vi "operationModeSelector.vi"() -> (6 "selectedMode":string, 7 "isError":bool, 8 "stopWaiting":bool)   [LabVIEW 2014]
panel:
  in  "ctrlDP":bool
  in  "ctrlManualForce":bool
  in  "ctrlManualThrusters":bool
  # "Please select an operational mode for CS Saucer"
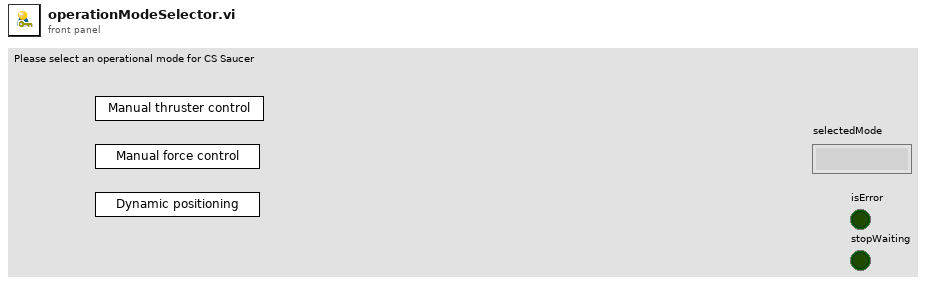
[diagram p1: front panel]
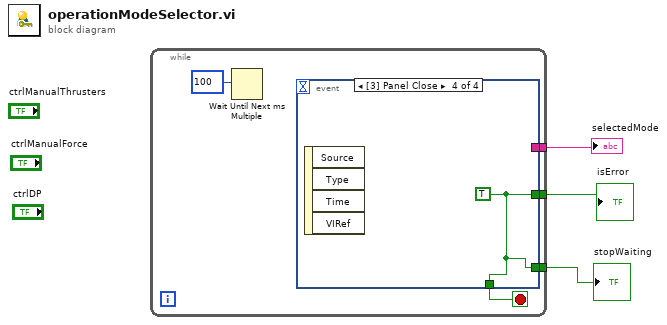
[diagram p0: block diagram]
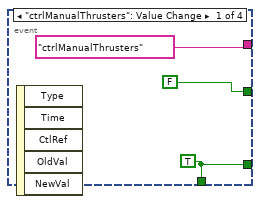
[diagram p2: hidden frame]
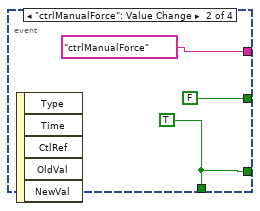
[diagram p3: hidden frame]
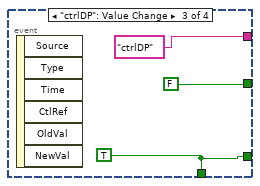
[diagram p4: hidden frame]
diagram:
  n1 = while {
    tunnel: [w8] -> w3
    tunnel: [w5] -> w2
    tunnel: [w4] -> w1
    stop <- w6 stop-if-true
    n2 = Wait Until Next ms Multiple(millisecond multiple=100) -> ()  [unwired: 1 out]
    n3 = event shown="[3] Panel Close" {
      selector: _ -> [_ _ _ _]
      dyn-events: _ -> [_ _ _ _]
      timeout: _ -> [_ _ _ _]
      tunnel: [w9 w12 w15 w18] -> w6
      tunnel: ["ctrlManualThrusters" "ctrlManualForce" "ctrlDP" _] -> w8
      tunnel: [FALSE FALSE FALSE w18] -> w5
      tunnel: [w9 w12 w15 w18] -> w4
      event "ctrlManualThrusters": Value Change {
        w9 = TRUE
        n4 = event-data() -> ()  [unwired: 6 out]
      }
      event "ctrlManualForce": Value Change {
        w12 = TRUE
        n5 = event-data() -> ()  [unwired: 6 out]
      }
      event "ctrlDP": Value Change {
        w15 = TRUE
        n6 = event-data() -> ()  [unwired: 7 out]
      }
      event Panel Close {
        w18 = TRUE
        n7 = event-data() -> ()  [unwired: 5 out]
      }
    }
  }
  "selectedMode" <- w3
  "isError" <- w2
  "stopWaiting" <- w1
